vi "join array jsons.vi"(8 "error in (no error)":errorcluster, 10 "jsons":string[](array[string]), 11 "Save Image in":refnum<class "Save Image.lvclass">) -> (0 "error out":errorcluster, 2 "concatenated json":string, 3 "Save Image out":refnum<class "Save Image.lvclass">)   [LabVIEW 2018, in "Save Image.lvclass"]
uses:
  Save Image.lvclass
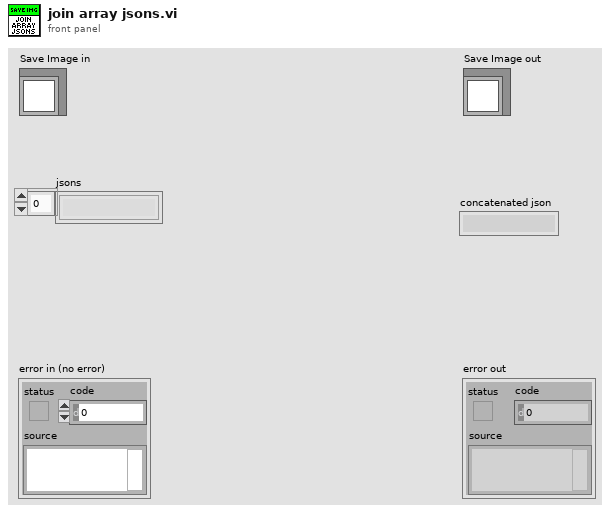
[diagram p1: front panel]
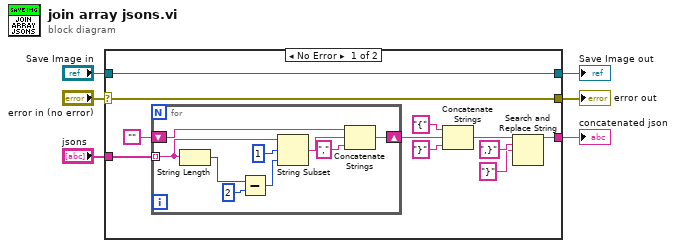
[diagram p0: block diagram]
diagram:
  n1 = case shown="No Error" "error in (no error)" {
    selector: "error in (no error)" -> [w16 w28]
    tunnel: [w16 w28] -> w5
    tunnel: [w17 w27] -> w3
    tunnel: "Save Image in" -> [w17 w27]
    tunnel: "jsons" -> [w11 _]
    tunnel: [w9 _] -> w1
    frame No Error {
      n2 = for {
        tunnel: w11 -> [w25] mode=indexing
        shift-right: [w24] -> w12
        shift-left: "" -> [w21]
        n3 = String Length(string=w25) -> (length=w20:i32)
        n4 = Subtract(x=w20, y=2) -> (x-y=w19:i32)
        n5 = String Subset(string=w25, offset (0)=1, length (rest)=w19) -> (substring=w23:string)
        n6 = Concatenate Strings(w21, w23, ",") -> (w24:string)
      }
      n7 = Concatenate Strings("{", w12, "}") -> (w10:string)
      n8 = Search and Replace String(input string=w10, search string=",}" ("substring (\"\")"), replace string="}" ("replace string (\"\")")) -> (result string=w9:string)  [unwired: 5 in, 3 out]
    }
    frame Error {
    }
  }
  "error out" <- w5
  "Save Image out" <- w3
  "concatenated json" <- w1
